vi "OFDM-SIM-Alamouti解码.vi"(2 "error in (no error)":errorcluster, 3 "信道2参数":cdb[][](array[numeric]) format="%#_6p", 4 "信道1参数":cdb[][](array[numeric]) format="%#_6p", 5 "信息符号":cdb[][](array[numeric]) format="%#_6p") -> (0 "error out":errorcluster, 1 "输出符号":cdb[](array[numeric]) format="%#_6p")   [LabVIEW 2018]
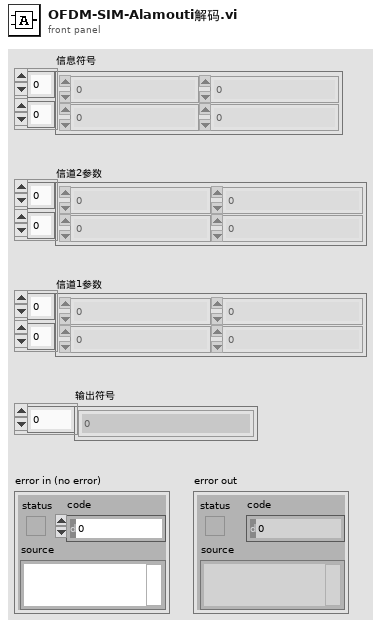
[diagram p1: front panel]
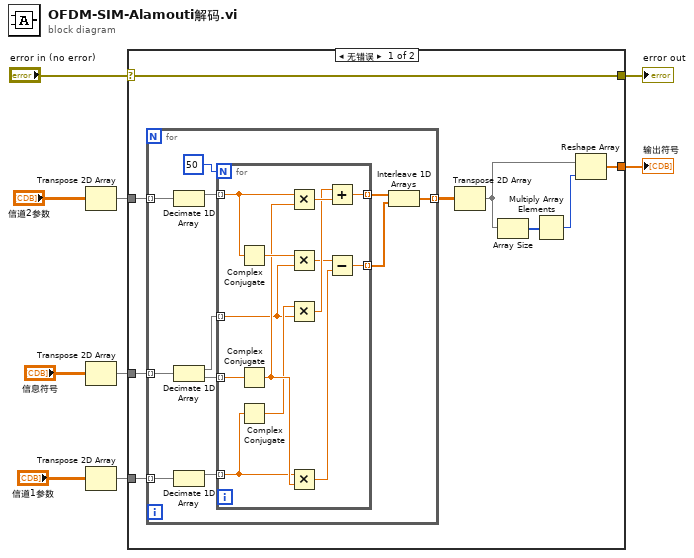
[diagram p0: block diagram]
diagram:
  n1 = Transpose 2D Array(2D array="信道2参数") -> (transposed array=w6:cdb[][])
  n2 = Transpose 2D Array(2D array="信息符号") -> (transposed array=w4:cdb[][])
  n3 = Transpose 2D Array(2D array="信道1参数") -> (transposed array=w1:cdb[][])
  n4 = case shown="无错误" "error in (no error)" {
    selector: "error in (no error)" -> [w18 w43]
    tunnel: [w18 w43] -> w8
    tunnel: w4 -> [w17 _]
    tunnel: w1 -> [w15 _]
    tunnel: w6 -> [w16 _]
    tunnel: [w13 _] -> w7
    frame No Error {
      n5 = for {
        tunnel: w17 -> [w28] mode=indexing
        tunnel: w16 -> [w21] mode=indexing
        tunnel: w15 -> [w27] mode=indexing
        tunnel: [w19] -> w14 mode=indexing
        n6 = Decimate 1D Array(w21) -> (w26:cdb[])  [unwired: 1 out]
        n7 = Decimate 1D Array(w28) -> (w29:cdb[], w24:cdb[])
        n8 = Decimate 1D Array(w27) -> (w25:cdb[])  [unwired: 1 out]
        n9 = for {
          N: 50 -> [_]
          tunnel: w26 -> [w34] mode=indexing
          tunnel: w29 -> [w33] mode=indexing
          tunnel: w25 -> [w35] mode=indexing
          tunnel: w24 -> [w32] mode=indexing
          tunnel: [w31] -> w23 mode=indexing
          tunnel: [w30] -> w22 mode=indexing
          n10 = Complex Conjugate(1:w34) -> (0:w40:cdb)
          n11 = Complex Conjugate(1:w32) -> (0:w39:cdb)
          n12 = Complex Conjugate(1:w35) -> (0:w36:cdb)
          n13 = Multiply(x=w34, y=w39) -> (x*y=w42:cdb)
          n14 = Multiply(x=w40, y=w33) -> (x*y=w38:cdb)
          n15 = Multiply(x=w36, y=w33) -> (x*y=w41:cdb)
          n16 = Multiply(x=w35, y=w39) -> (x*y=w37:cdb)
          n17 = Add(x=w41, y=w42) -> (x+y=w31:cdb)
          n18 = Subtract(x=w38, y=w37) -> (x-y=w30:cdb)
        }
        n19 = Interleave 1D Arrays ("交织一维数组")(w23, w22) -> (w19:cdb[])
      }
      n20 = Transpose 2D Array(2D array=w14) -> (transposed array=w10:cdb[][])
      n21 = Array Size(array=w10) -> (size(s)=w11:i32[])
      n22 = Multiply Array Elements(1:w11) -> (0:w12:i32)
      n23 = Reshape Array(w10, w12) -> (w13:cdb[])
    }
    frame Error {
    }
  }
  "error out" <- w8
  "输出符号" <- w7
